vi "String Constant - One Line State String Unwired.vi"   [LabVIEW 2013]
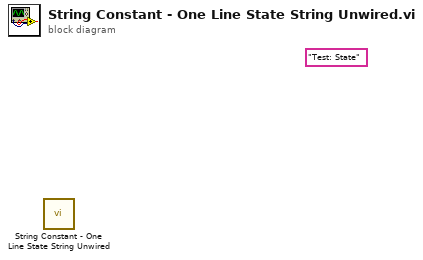
[diagram p0: block diagram]
diagram:
  (unwired) "Test: State"
  n1 = call "String Constant - One Line State String Unwired.vi"() -> ()  [unwired: 12 in]
